vi "STRUCT_1_STAGE.vi"(8 "Dataflow In":errorcluster) -> (0 "Dataflow Out":errorcluster)   [LabVIEW 2019]
panel:
  # "*******************************************************************\nBiogas Plant Control\n\nAuthor: Paul Zügel\nGCSC-Frankfurt am Main 2020\n\n*******************************************************************"
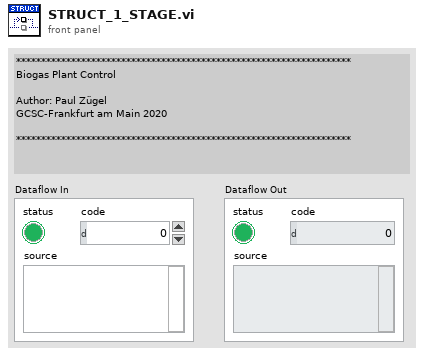
[diagram p1: front panel]
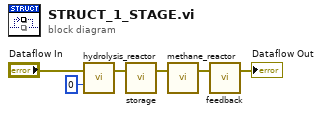
[diagram p0: block diagram]
diagram:
  n1 = call "hydrolysis_reactor.vi"("#"=i16 0, "Dataflow In"="Dataflow In") -> ("Dataflow Out"=w6:errorcluster)  [unwired: 2 in]
  n2 = call "storage.vi"("Dataflow In #1"=w6) -> ("Dataflow Out"=w5:errorcluster)  [unwired: 3 in]
  n3 = call "methane_reactor.vi"("Dataflow In"=w5) -> ("Dataflow Out"=w4:errorcluster)  [unwired: 2 in]
  n4 = call "feedback.vi"("Dataflow In"=w4) -> ("Dataflow Out"=→"Dataflow Out":errorcluster)  [unwired: 2 in]
